vi "UTF-8 String Probe.vi"(1 "UTF-8":refnum<class "UTF-8 String.lvclass">) -> (0 "Boolean":bool)   [LabVIEW 2020, in "G-Unicode.lvlib" / "UTF-8 String.lvclass"]
uses:
  UTF-8 String.lvclass
  UTF-8 String.lvclass/UTF-8 String.ctl
  G-Unicode.lvlib
panel:
  out "Unicode":string
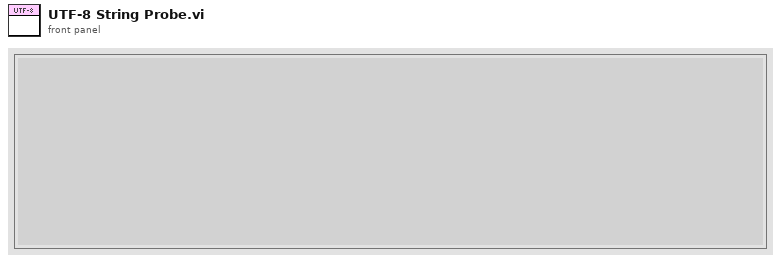
[diagram p1: front panel]
types:
  T1 = typedef "G-Unicode.lvlib/Encoded UTF-8 String.ctl" = string
  T2 = typedef "G-Unicode.lvlib/Encoded UTF-16LE String.ctl" = string
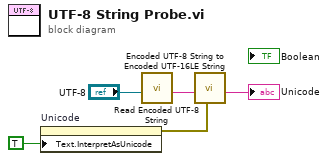
[diagram p0: block diagram]
diagram:
  n1 = property on="Unicode" class="Str"("Text.InterpretAsUnicode"=TRUE ("Force Unicode Text")) -> (error out=w1:errorcluster)  [unwired: 2 in, 1 out]
  n2 = call "Read Encoded UTF-8 String.vi"("UTF-8 String"="UTF-8") -> ("Encoded UTF-8 String"=w3:T1)  [unwired: 10 in]
  n3 = call "Encoded UTF-8 String to Encoded UTF-16LE String.vi"("error in"=w1, "Encoded UTF-8 String"=w3) -> ("Encoded UTF-16LE String"=→"Unicode":T2)  [unwired: 8 in, 1 out]
